vi "Enter Leonardo Bootloader.vi"(8 "Error In":errorcluster, 11 "VISA resource name":refnum<visa-resource-name>) -> (0 "Error Out":errorcluster, 2 "Found?":bool, 3 "VISA resource name":refnum<visa-resource-name>)   [LabVIEW 2020, in "LMH-LINX.lvlib"]
uses:
  LMH-LINX.lvlib
  <vilib>/Instr/_visa.llb/VISA Configure Serial Port (Instr).vi
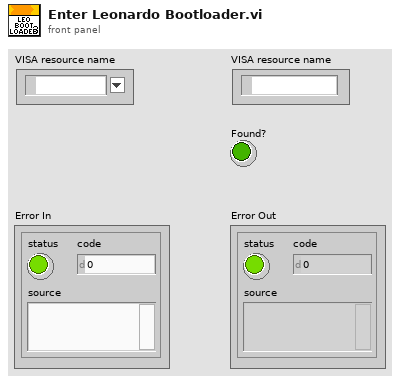
[diagram p1: front panel]
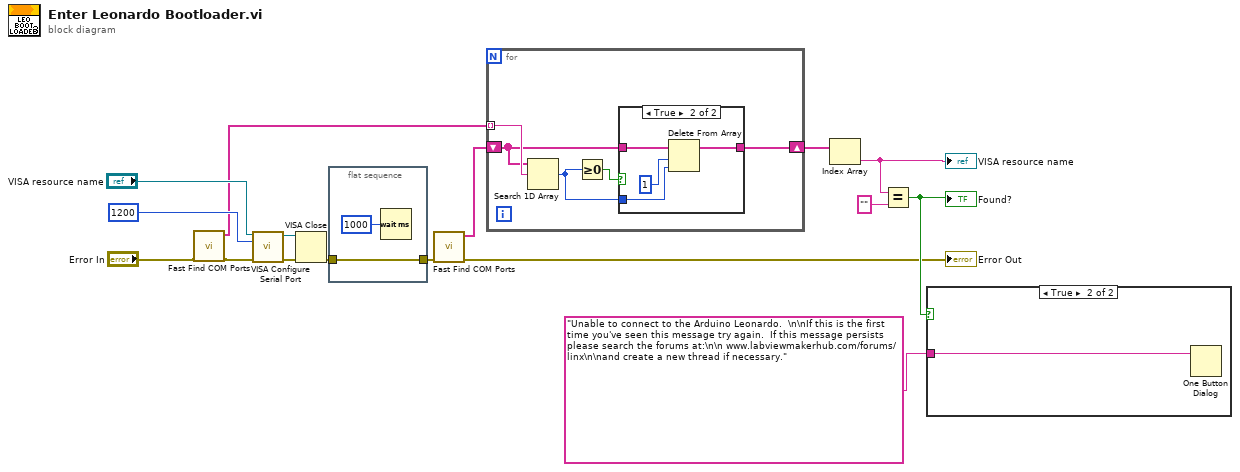
[diagram p0: block diagram]
diagram:
  n1 = call "Fast Find COM Ports.vi"("Error In"="Error In") -> ("Error Out"=w7:errorcluster, "COM Ports"=w6:string[])  [unwired: 9 in]
  n2 = call-poly "VISA Configure Serial Port"("VISA resource name"="VISA resource name", "baud rate (9600)"=u32 1200, "error in (no error)"=w7) -> ("VISA resource name out"=w13:refnum<visa-resource-name>, "error out"=w14:errorcluster)  [unwired: 11 in]
  n3 = VISA Close(VISA resource name=w13, error in (no error)=w14) -> (error out=w2:errorcluster)
  n4 = flat-sequence {
    tunnel: [w18] -> w3
    tunnel: w2 -> [w18]
    frame #0 {
      n5 = Wait (ms)(milliseconds to wait=u32 1000) -> ()  [unwired: 1 out]
    }
  }
  n6 = call "Fast Find COM Ports.vi"("Error In"=w3) -> ("Error Out"=→"Error Out":errorcluster, "COM Ports"=w4:string[])  [unwired: 9 in]
  n7 = for {
    tunnel: w6 -> [w23] mode=indexing
    shift-right: [w22] -> w12
    shift-left: w4 -> [w21]
    n8 = Search 1D Array(1D array=w21, element=w23) -> (index of element=w20:i32)  [unwired: 1 in]
    n9 = Greater Or Equal To 0?(x=w20) -> (x >= 0?=w19:bool)
    n10 = case shown="True" w19 {
      tunnel: [w24 w28] -> w22
      tunnel: w21 -> [w24 w27]
      tunnel: w20 -> [_ w25]
      frame False {
      }
      frame True {
        n11 = Delete From Array(array=w27, length=1, index=w25) -> (array with subset deleted=w28:string[])  [unwired: 1 out]
      }
    }
  }
  n12 = Index Array(array=w12) -> (element=w9:string)  [unwired: 1 in]
  "VISA resource name" <- w9
  n13 = Equal?(x=w9, y="") -> (x = y?=w10:bool)
  "Found?" <- w10
  n14 = case shown="True" w10 {
    tunnel: "Unable to connect to the Arduino Leonardo.  \n\nIf this is the first time you've seen this message try again.  If this message persists please search the forums at:\n\n www.labviewmakerhub.com/forums/linx\n\nand create a new thread if necessary." ("message") -> [_ w29]
    frame False {
    }
    frame True {
      n15 = One Button Dialog(message=w29) -> ()  [unwired: 1 in, 1 out]
    }
  }
